vi "Pregunta Tipo.vi"(8 "error in (no error)":errorcluster, 11 "Vehiculo de Motor in":refnum<class "Vehiculo de Motor.lvclass">) -> (0 "error out":errorcluster, 3 "Vehiculo de Motor out":refnum<class "Vehiculo de Motor.lvclass">)   [LabVIEW 2020, in "Vehiculo de Motor.lvclass"]
uses:
  Vehiculo de Motor.lvclass
  Vehiculo de Motor.lvclass/Vehiculo de Motor.ctl
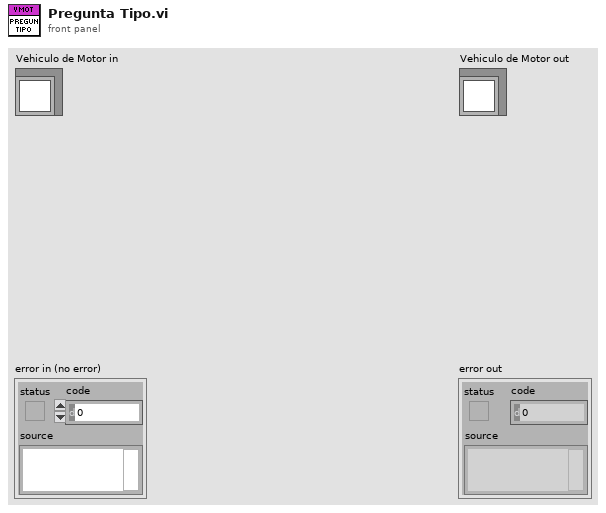
[diagram p1: front panel]
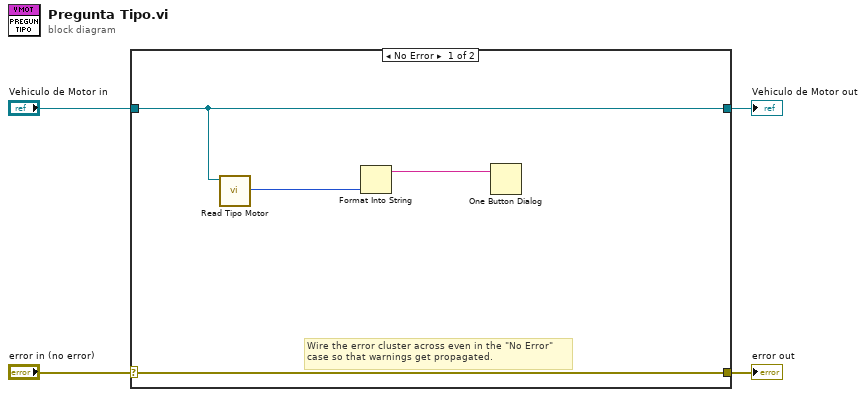
[diagram p0: block diagram]
diagram:
  n1 = case shown="No Error" "error in (no error)" {
    selector: "error in (no error)" -> [w8 w10]
    tunnel: [w8 w10] -> w3
    tunnel: [w7 w9] -> w1
    tunnel: "Vehiculo de Motor in" -> [w7 w9]
    frame No Error {
      # "Wire the error cluster across even in the \"No Error\"\ncase so that warnings get propagated."
      n2 = call "Read Tipo Motor.vi"("Vehiculo de Motor in"=w7) -> ("Tipo Motor"=w6:enum16{"Eléctrico", "Gasolina"})  [unwired: 8 in, 2 out]
      n3 = Format Into String(w6) -> (resulting string=w5:string)  [unwired: 3 in, 1 out]
      n4 = One Button Dialog(message=w5) -> ()  [unwired: 1 in, 1 out]
    }
    frame Error {
    }
  }
  "error out" <- w3
  "Vehiculo de Motor out" <- w1
